vi "Write to Text Log File.vi"(6 "Data":dbl[][](array[numeric]), 8 "error in (no error)":errorcluster, 9 "Channel Names in":string[](array[string]), 10 "Group Names in":string[](array[string]), 11 "Text Log File in":refnum<class "Text Log File.lvclass">) -> (0 "error out":errorcluster, 3 "Text Log File out":refnum<class "Text Log File.lvclass">)   [LabVIEW 2015, in "Text Log File.lvclass"]
doc: "Writes data to the text file using the specified delimiter and format string. The channel and group names are ignored. The header for the file should be written in advance using Write Log Header.vi."
uses:
  Text Log File.lvclass
  Text Log File.lvclass/Text Log File.ctl
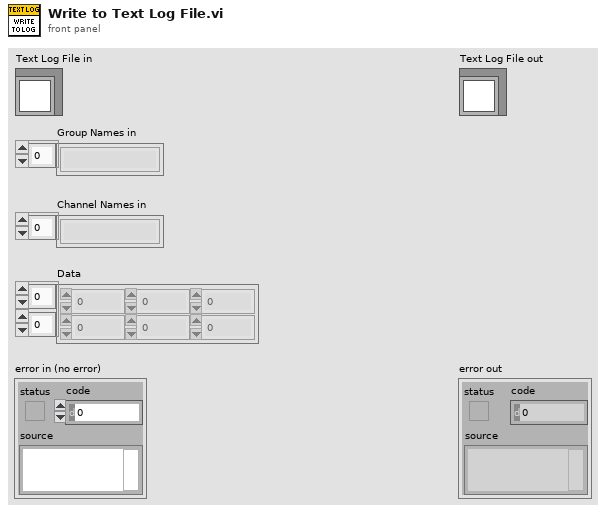
[diagram p1: front panel]
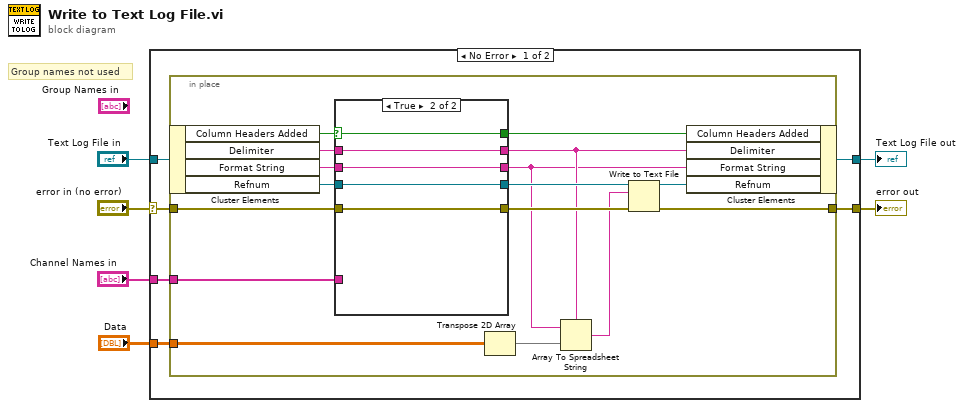
[diagram p0: block diagram]
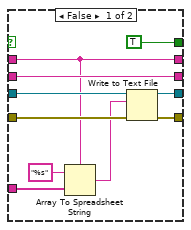
[diagram p2: hidden frame]
diagram:
  # "Group names not used"
  n1 = case shown="No Error" "error in (no error)" {
    selector: "error in (no error)" -> [w8 w44]
    tunnel: [w12 w45] -> w6
    tunnel: "Data" -> [w11 _]
    tunnel: [w10 w44] -> w4
    tunnel: "Text Log File in" -> [w9 w45]
    tunnel: "Channel Names in" -> [w7 _]
    frame No Error {
      n2 = in-place {
        in-place-border: w8 -> [w21]
        in-place-border: w11 -> [w27]
        in-place-border: [w26] -> w10
        in-place-border: w7 -> [w22]
        n3 = in-place-cluster #1(w9) -> ("Column Headers Added"=w16:bool, "Delimiter"=w19:string, "Format String"=w17:string, "Refnum"=w14:refnum<file>)
        n4 = case shown="True" w16 {
          selector: w16 -> [_ w43]
          tunnel: [w38 w41] -> w28
          tunnel: w14 -> [w36 w42]
          tunnel: [w35 w42] -> w23
          tunnel: [TRUE w43] -> w15
          tunnel: w22 -> [w34 _]
          tunnel: w21 -> [w33 w41]
          tunnel: [w29 w40] -> w20
          tunnel: w19 -> [w29 w40]
          tunnel: [w30 w39] -> w18
          tunnel: w17 -> [w30 w39]
          frame False {
            n5 = Array To Spreadsheet String(delimiter (Tab)=w29, array=w34, 3:"%s" ("format string")) -> (spreadsheet string=w31:string)
            n6 = Write to Text File(file (use dialog)=w36, text=w31, error in=w33) -> (refnum out=w35:refnum<file>, error out=w38:errorcluster)  [unwired: 1 in, 1 out]
          }
          frame True {
          }
        }
        n7 = Transpose 2D Array(2D array=w27) -> (transposed array=w25:dbl[][])
        n8 = Array To Spreadsheet String(delimiter (Tab)=w20, array=w25, 3:w18) -> (spreadsheet string=w24:string)
        n9 = Write to Text File(file (use dialog)=w23, text=w24, error in=w28) -> (refnum out=w13:refnum<file>, error out=w26:errorcluster)  [unwired: 1 in, 1 out]
        n10 = in-place-cluster #1("Column Headers Added"=w15, "Delimiter"=w20, "Format String"=w18, "Refnum"=w13) -> (w12:refnum<class "Text Log File.lvclass">)
      }
    }
    frame Error {
    }
  }
  "error out" <- w4
  "Text Log File out" <- w6
